vi "SVX Polar Plot.vi"   [LabVIEW 2017, in "SoundVib_OAVisualization.lvlib"]
doc: "Prepares polar plot data for displaying on a Polar Plot. Use this VI to show magnitude versus phase for a specific order. Wire data to the <B>magnitudes [RMS]</B> and <B>phases [phase lag]</B> inputs to determine the polymorphic instance to use or manually select the instance."
uses:
  <vilib>/addons/Sound and Vibration/Order Analysis/Data Presentation/SoundVib_OAVisualization.lvlib
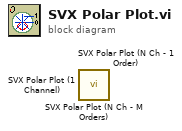
[diagram p0: block diagram]
diagram:
  n1 = call <vilib>:"SVX Polar Plot (N Ch - M Orders).vi"() -> ()  [unwired: 13 in, 3 out]
  n2 = call <vilib>:"SVX Polar Plot (N Ch - 1 Order).vi"() -> ()  [unwired: 13 in, 3 out]
  n3 = call <vilib>:"SVX Polar Plot (1 Channel).vi"() -> ()  [unwired: 13 in, 3 out]
